vi "Insert_PKYK.vi"(8 "error in (no error)":errorcluster, 10 "PokaYoke Parameter":T1 {"MachineCode" items=["MCIG", "MCPC", "MCSA", "MCCA", "MCAC", "MCLA", "MCCM", "MCSC", "MCPA", "MCLP", "MCHP", "MCBC", "MCFA", "MCSR", "MCFV"]; "ExpiryDate" format="%<%I:%M:%S%3u %p\n%d-%m-%Y>T"; "EntDt" format="%<%I:%M:%S%3u %p\n%d-%m-%Y>T"; "UpdDt" format="%<%I:%M:%S%3u %p\n%d-%m-%Y>T"}, 11 "Refnum in":T6) -> (0 "error out":errorcluster, 3 "Refnum out":T6)   [LabVIEW 2020]
uses:
  <vilib>/addons/database/Connection.llb/Conn ObjectReference.ctl
  Controls/Line_PKYK.ctl
  Controls/PARA_CONTROL_STR.ctl
  Controls/PKYK_MCODE.ctl
  Controls/PKYK_DATE.ctl
  Controls/PKYK_Result.ctl
  <vilib>/addons/database/NI_Database_API.lvlib
panel:
  out "resulting string":string
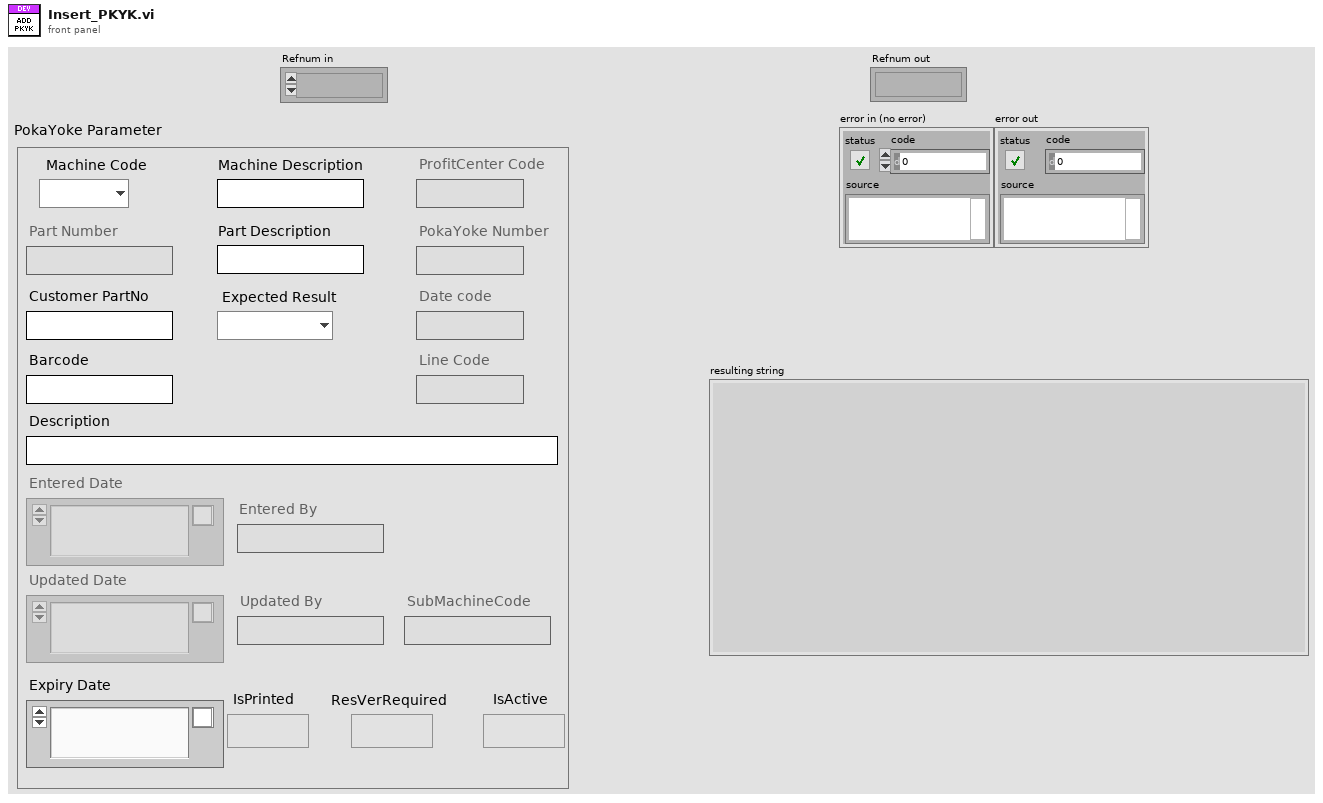
[diagram p1: front panel]
types:
  T1 = typedef "Line_PKYK.ctl" = cluster{"ProfitCenterCode":string, "LineCode":string, "Datecode":string, "PartNumber":T2, "PartDescription":T2, "CustPartNo":T2, "MachineCode":T3, "MachineDescription":T2, "PokaYokeNumber":string, "Description":string, "ExpiryDate":T4, "Barcode":T2, "IsPrinted":bool, "IsActive":bool, "EntBy":T2, "EntDt":T4, "UpdBy":T2, "UpdDt":T4, "ExpResult":T5, "ResVerRequired":bool, "SubMachineCode":T2}
  T2 = typedef "PARA_CONTROL_STR.ctl" = string
  T3 = typedef "PKYK_MCODE.ctl" = u16
  T4 = typedef "PKYK_DATE.ctl" = timestamp
  T5 = typedef "PKYK_Result.ctl" = enum16{"FAIL", "PASS"}
  T6 = typedef "NI_Database_API.lvlib/Conn ObjectReference.ctl" = refnum<k1>
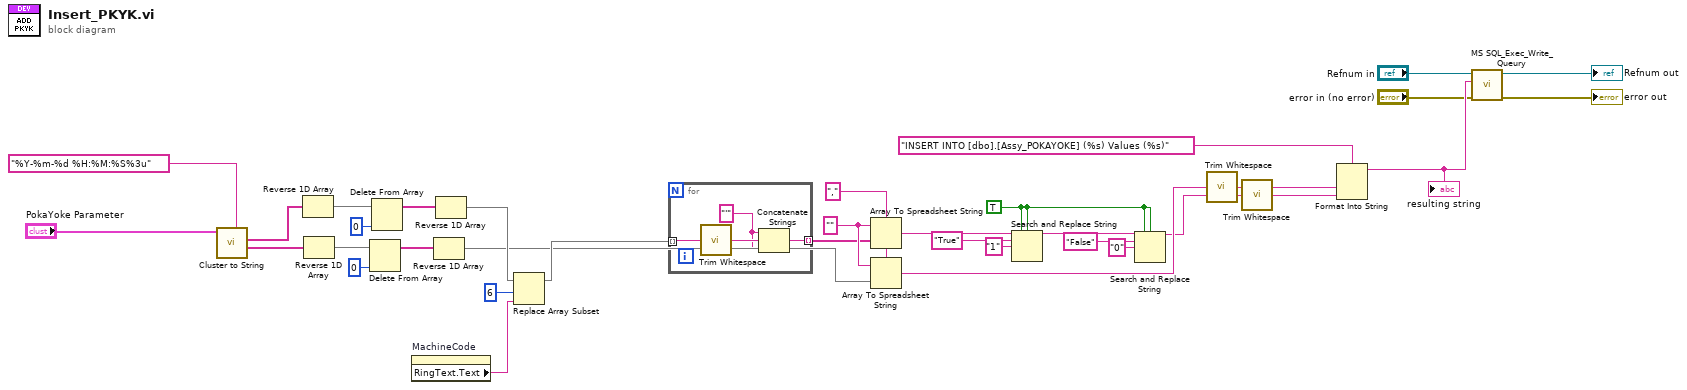
[diagram p0: block diagram]
diagram:
  w28 = TRUE ("replace all? (F)")
  w34 = "," ("delimiter (Tab)")
  w33 = "" ("format string")
  n1 = call <userlib>:"Cluster to String.vi"("Time Format String"="%Y-%m-%d %H:%M:%S%3u" ("time format string (%c)"), "Variant In"="PokaYoke Parameter") -> ("Format String Name"=w4:string[], "Format String Array"=w12:string[])  [unwired: 6 in, 2 out]
  n2 = Reverse 1D Array(array=w12) -> (reversed array=w11:string[])
  n3 = Reverse 1D Array(array=w4) -> (reversed array=w5:string[])
  n4 = Delete From Array(array=w5, index=0) -> (array with subset deleted=w7:string[])  [unwired: 1 in, 1 out]
  n5 = Delete From Array(array=w11, index=0) -> (array with subset deleted=w9:string[])  [unwired: 1 in, 1 out]
  n6 = property on="MachineCode" class="Ring (strict)"() -> ("RingText.Text"=w15:string)  [unwired: 2 in, 2 out]
  n7 = Reverse 1D Array(array=w7) -> (reversed array=w3:string[])
  n8 = Reverse 1D Array(array=w9) -> (reversed array=w8:string[])
  n9 = Replace Array Subset(array=w8, new element=w15, index=6) -> (w13:string[])
  n10 = for {
    tunnel: w13 -> [w39] mode=indexing
    tunnel: [w36] -> w14 mode=indexing
    w37 = "'" ("string")
    n11 = call <vilib>:"Trim Whitespace.vi"("string"=w39) -> ("trimmed string"=w38:string)  [unwired: 1 in]
    n12 = Concatenate Strings(w37, w38, w37) -> (w36:string)
  }
  n13 = Array To Spreadsheet String(delimiter (Tab)=w34, array=w14, 3:w33) -> (spreadsheet string=w25:string)
  n14 = Array To Spreadsheet String(delimiter (Tab)=w34, array=w3, 3:w33) -> (spreadsheet string=w23:string)
  n15 = Search and Replace String(replace all?=w28, case sensitive?=w28, input string=w25, search string="True", replace string="1" ("replace string (\"\")")) -> (result string=w29:string)  [unwired: 3 in, 3 out]
  n16 = Search and Replace String(replace all?=w28, case sensitive?=w28, input string=w29, search string="False", replace string="0" ("replace string (\"\")")) -> (result string=w22:string)  [unwired: 3 in, 3 out]
  n17 = call <vilib>:"Trim Whitespace.vi"("string"=w23) -> ("trimmed string"=w2:string)  [unwired: 1 in]
  n18 = call <vilib>:"Trim Whitespace.vi"("string"=w22) -> ("trimmed string"=w1:string)  [unwired: 1 in]
  n19 = Format Into String(format string="INSERT INTO [dbo].[Assy_POKAYOKE] (%s) Values (%s)", w2, w1) -> (resulting string=w21:string)  [unwired: 2 in, 1 out]
  "resulting string" <- w21
  n20 = call "MS SQL_Exec_Write_Queury.vi"("error in (no error)"="error in (no error)", "Query"=w21, "Refnum in"="Refnum in") -> ("error out"=→"error out":errorcluster, "Refnum out"=→"Refnum out":T6)  [unwired: 7 in]
